vi "main.vi"() -> ()   [LabVIEW 2015]
uses:
  LabviewSubVI/RFConfig/RF_Config.ctl
  LabviewSubVI/RFConfig/StudentMsg.ctl
panel:
  out "信宿数据":dbl[](graph)
  out "信源数据":dbl[](graph)
  out "时隙同步相关峰":dbl[](graph)
  in  "相位纠正开关":enum16{"关", "开"}(ring)=enum."开"
  in  "载波调制开关":enum16{"关", "开"}(ring)=enum."开"
  in  "信道编码开关":enum16{"关", "开"}(ring)=enum."开"
  in  "解调载波初相位":enum16{"0", "180"}(ring) caption="下拉列表"
  in  "信噪比(dB)":dbl=40.0 caption="crc_num" min=-20.0 max=40.0 step=0.1 format="%#_13g"
  out "误码率":dbl format="%#_4g"
  out "误码数":dbl format="%#_13g"
  out "CRC\n校验结果":bool[](array[boolean])
  out "接收信号波形":dbl[](graph)
  in  "pcip":string="192.168.1.180"
  in  "xsrpip":string="192.168.1.166"
  out "发送信号波形":dbl[](graph)
  in  "运行方式":enum16{"仿真系统", "真实系统"}(ring)
  in  "?":T1={"发射频率"=2000000000, "发射衰减"=30, "接收频率"=2000000000, "接收增益"=22, "接收通道"=enum."RxCh1", "发射通道"=enum."TxCh1"} {"接收增益" max=40 format="%.0fdB"; "接收频率" min=70000000 max=6000000000 format="%.6pHz"; "发射衰减" max=90 format="%.0fdB"; "发射频率" min=70000000 max=6000000000 format="%.6pHz"}
  out "实验学生信息":T2={"姓名"="XXX\n", "学号"="XXX", "班级"="XXX", "学校"="XXX"}
  # "基于XSRP软件无线电平台的BPSK数字调制通信系统"
  # "实验参数设置"
  # "实验学生信息"
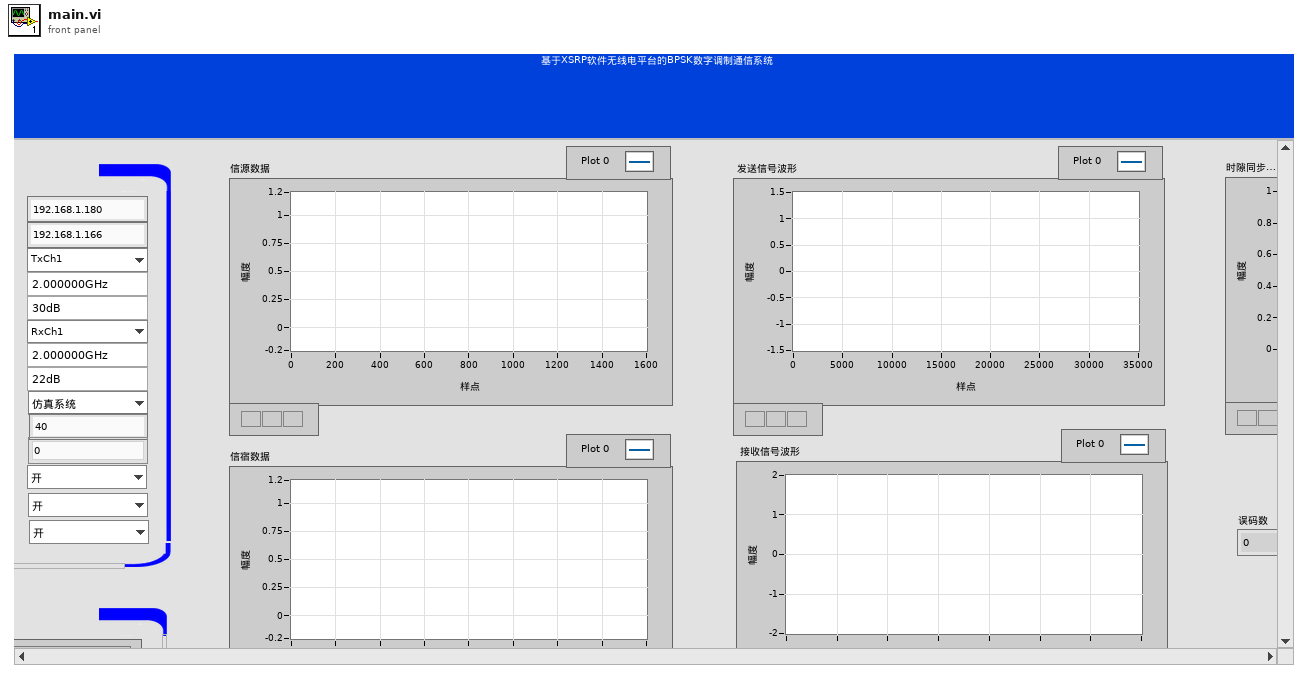
[diagram p1: front panel]
types:
  T1 = typedef "RF_Config.ctl" = cluster{"发射频率":u64, "发射衰减":u8, "接收频率":u64, "接收增益":u8, "接收通道":enum16{"RxCh1", "RxCh2"}, "发射通道":enum16{"TxCh1", "TxCh2"}}
  T2 = typedef "StudentMsg.ctl" = cluster{"姓名":string, "学号":string, "班级":string, "学校":string}
  T3 = enum8{"Enabled", "Disabled", "Disabled and Grayed Out"}
  T4 = cluster{"接收通道":enum16{"RxCh1", "RxCh2"}, "接收频率":u32, "接收增益":u8}
  T5 = cluster{"发射通道":enum16{"TxCh1", "TxCh2"}, "发射频率":u32, "发射衰减":u8}
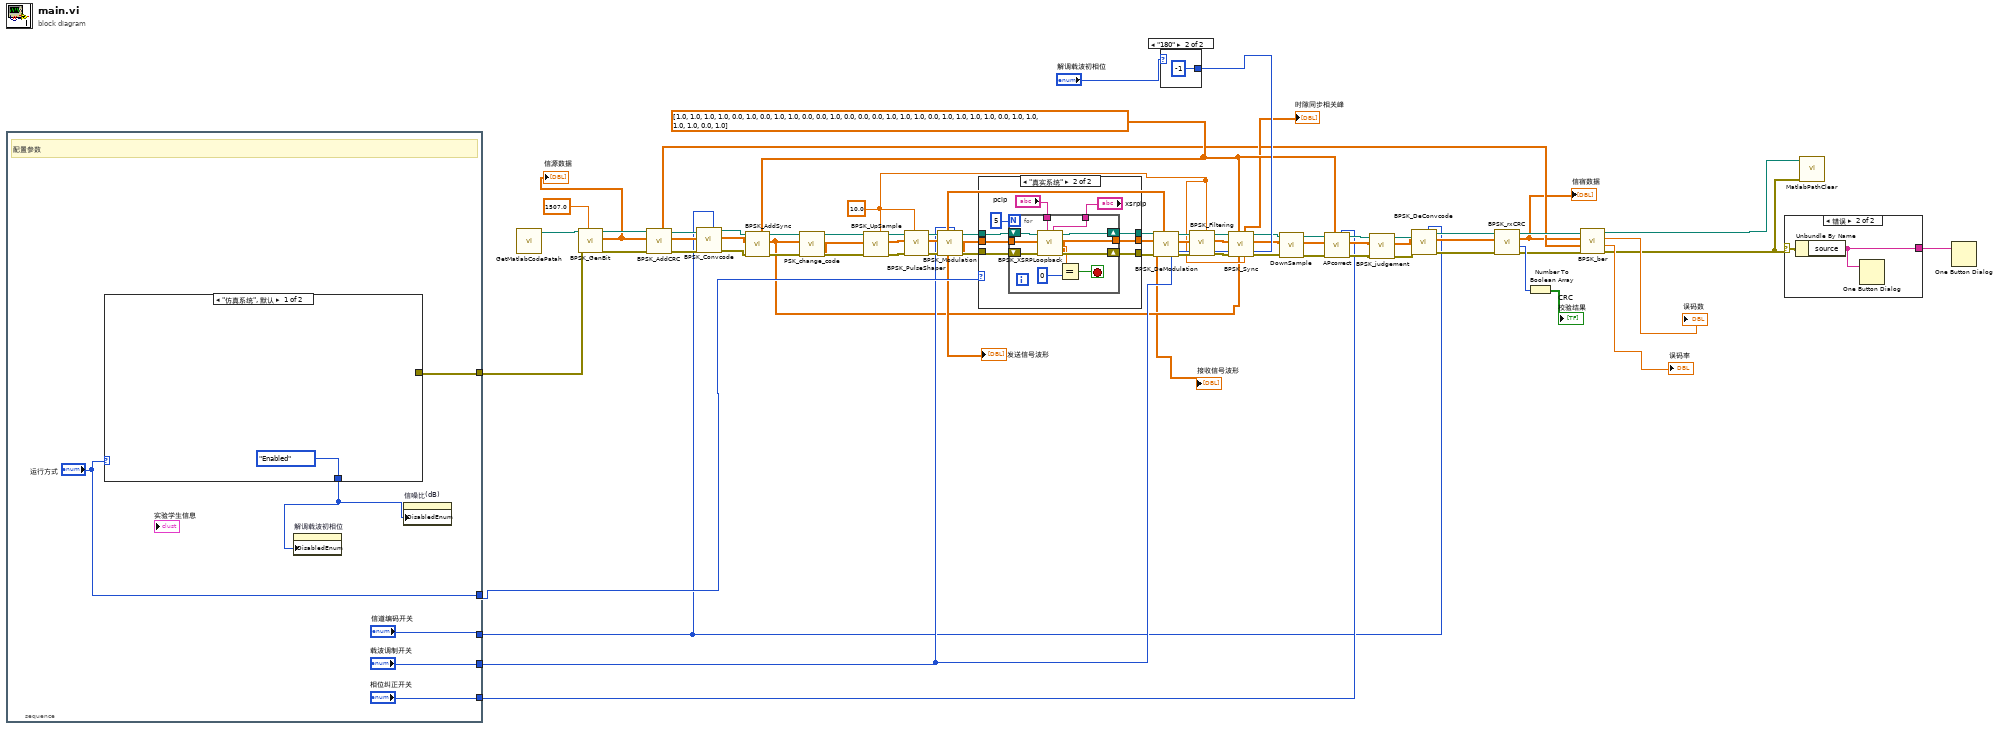
[diagram p0: block diagram]
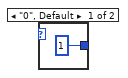
[diagram p2: hidden frame]
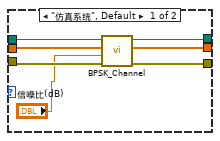
[diagram p3: hidden frame]
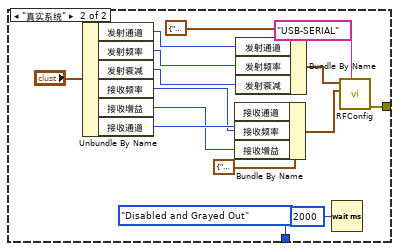
[diagram p4: hidden frame]
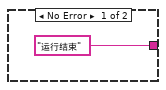
[diagram p5: hidden frame]
diagram:
  w8 = 10.0 ("UpSampleRate")
  w12 = dbl[] [1.0, 1.0, 1.0, 1.0, 0.0, 1.0, 0.0, 1.0, 1.0, 0.0, 0.0, 1.0, 0.0, 0.0, 0.0, 1.0, 1.0, 1.0, 0.0, 1.0, 1.0, 1.0, 1.0, 0.0, 1.0, 1.0, 1.0, 1.0, 0.0, 1.0] ("1-D Array of Real")
  n1 = stacked-sequence {
    tunnel: [w77] -> w33
    tunnel: ["运行方式"] -> w44
    tunnel: ["信道编码开关"] -> w9
    tunnel: ["载波调制开关"] -> w11
    tunnel: ["相位纠正开关"] -> w10
    frame #0 {
      # "配置参数"
      n2 = case shown="\"仿真系统\", 默认" "运行方式" {
        tunnel: [_ w82] -> w77
        tunnel: [T3."Enabled" ("Disabled") T3."Disabled and Grayed Out" ("Disabled")] -> w75
        frame "仿真系统", Default {
        }
        frame "真实系统" {
          n3 = Unbundle By Name("?") -> ("发射通道"=w90:enum16{"TxCh1", "TxCh2"}, "发射频率"=w89:u64, "发射衰减"=w88:u8, "接收频率"=w84:u64, "接收增益"=w85:u8, "接收通道"=w86:enum16{"RxCh1", "RxCh2"})
          n4 = Bundle By Name(cluster=T4 {"接收通道"=enum."RxCh1", "接收频率"=0, "接收增益"=0} ("接收参数设置"), "接收通道"=w86, "接收频率"=w84, "接收增益"=w85) -> (w83:T4)
          n5 = Bundle By Name(cluster=T5 {"发射通道"=enum."TxCh1", "发射频率"=0, "发射衰减"=0} ("发射参数设置"), "发射通道"=w90, "发射频率"=w89, "发射衰减"=w88) -> (w92:T5)
          n6 = Wait (ms)(milliseconds to wait=u32 2000) -> ()  [unwired: 1 out]
          n7 = call "RFConfig.vi"("USB-SERIAL name"="USB-SERIAL", "接收参数设置"=w83, "发射参数设置"=w92) -> ("error out"=w82:errorcluster)  [unwired: 8 in]
        }
      }
      n8 = property on="解调载波初相位" class="Enum (严格)"("DisabledEnum"=w75) -> ()  [unwired: 2 in, 2 out]
      n9 = property on="信噪比(dB)" class="DigNum (严格)"("DisabledEnum"=w75) -> ()  [unwired: 2 in, 2 out]
    }
  }
  n10 = call "GetMatlabCodePatah.vi"() -> ("MatlabCodePath"=w47:path)  [unwired: 11 in]
  n11 = call "BPSK_GenBit.vi"("MsgLen"=1507.0, "error in (no error)"=w33, "PathIn"=w47) -> ("error out"=w45:errorcluster, "SendBit"=w5:dbl[], "PathOut"=w46:path)  [unwired: 6 in]
  "信源数据" <- w5
  n12 = call "BPSK_AddCRC.vi"("error in (no error)"=w45, "input_data"=w5, "PathIn"=w46) -> ("error out"=w69:errorcluster, "output_data"=w68:dbl[], "PathOut"=w70:path)  [unwired: 6 in]
  n13 = call "BPSK_Convcode.vi"("EN_Convcode"=w9, "error in"=w69, "input_data"=w68, "Path In"=w70) -> ("error out"=w26:errorcluster, "output_data"=w25:dbl[], "Path Out"=w31:path)  [unwired: 5 in]
  n14 = call "BPSK_AddSync.vi"("Preamble"=w12, "error in (no error)"=w26, "Channel_Bit"=w25, "PathIn"=w31) -> ("error out"=w27:errorcluster, "data"=w3:dbl[], "PathOut"=w30:path)  [unwired: 5 in]
  n15 = call "PSK_change_code.vi"("error in (no error)"=w27, "input_data"=w3, "PathIn"=w30) -> ("error out"=w28:errorcluster, "PathOut"=w29:path, "x"=w6:dbl[])  [unwired: 6 in]
  n16 = call "BPSK_UpSample.vi"("UpSampleRate"=w8, "error in (no error)"=w28, "input_data"=w6, "PathIn"=w29) -> ("error out"=w57:errorcluster, "output_data"=w2:dbl[], "PathOut"=w58:path)  [unwired: 5 in]
  n17 = call "BPSK_PulseShaper.vi"("UpSampleRate"=w8, "error in (no error)"=w57, "input_data"=w2, "PathIn"=w58) -> ("error out"=w56:errorcluster, "out_data"=w34:dbl[], "PathOut"=w55:path)  [unwired: 5 in]
  n18 = call "BPSK_Modulation.vi"("EN_Modulation"=w11, "error in (no error)"=w56, "input_data"=w34, "PathIn"=w55) -> ("error out"=w53:errorcluster, "PathOut"=w54:path, "output_data"=w35:dbl[], "y"=w36:dbl[])  [unwired: 4 in]
  "发送信号波形" <- w35
  n19 = case shown="\"真实系统\"" w44 {
    tunnel: w54 -> [w98 w106]
    tunnel: w35 -> [w100 w102]
    tunnel: w53 -> [w99 w107]
    tunnel: [w97 w105] -> w52
    tunnel: [w96 w101] -> w1
    tunnel: [w95 w104] -> w51
    frame "仿真系统", Default {
      n20 = call "BPSK_Channel.vi"("error in (no error)"=w99, "snr"="信噪比(dB)", "txSig"=w100, "PathIn"=w98) -> ("error out"=w95:errorcluster, "rxSig"=w96:dbl[], "PathOut"=w97:path)  [unwired: 5 in]
    }
    frame "真实系统" {
      n21 = for {
        N: 5 -> [_]
        tunnel: "pcip" -> [w120]
        tunnel: "xsrpip" -> [w119]
        tunnel: [w110] -> w101
        shift-right: [w116] -> w104
        shift-left: w107 -> [w112]
        shift-right: [w117] -> w105
        shift-left: w106 -> [w118]
        tunnel: w102 -> [w111]
        stop <- w113 stop-if-true
        n22 = call "BPSK_XSRPLoopback.vi"("tx_data"=w111, "xsrpip"=w119, "pcip"=w120, "error in (no error)"=w112, "PathIn"=w118) -> ("error out"=w116:errorcluster, "ERR_CODE"=w114:dbl, "PathOut"=w117:path, "rxdataIQ"=w110:cdb[])  [unwired: 3 in]
        n23 = Equal?(x=w114, y=0) -> (x = y?=w113:bool)
      }
    }
  }
  "接收信号波形" <- w1
  n24 = case shown="\"180\"" "解调载波初相位" {
    tunnel: [1 -1] -> w38
    frame "0", Default {
    }
    frame "180" {
    }
  }
  n25 = call "BPSK_DeModulation.vi"("input_data"=w1, ",EN_Modulation"=w11, "ini_pha"=w38, "y"=w36, "error in (no error)"=w51, "PathIn"=w52) -> ("error out"=w50:errorcluster, "re_data"=w48:dbl[], "PathOut"=w49:path)  [unwired: 3 in]
  n26 = call "BPSK_Filtering.vi"("UpSampleRate"=w8, "error in (no error)"=w50, "input_data"=w48, "PathIn"=w49) -> ("error out"=w65:errorcluster, "out_data"=w66:dbl[], "PathOut"=w67:path)  [unwired: 5 in]
  n27 = call "BPSK_Sync.vi"("UpSampleRate"=w8, "data"=w3, "Preamble"=w12, "error in (no error)"=w65, "input_data"=w66, "PathIn"=w67) -> ("error out"=w18:errorcluster, "output_data"=w19:dbl[], "PathOut"=w22:path, "RecvCorr"=→"时隙同步相关峰":dbl[])  [unwired: 2 in]
  n28 = call "DownSample.vi"("error in (no error)"=w18, "input_data"=w19, "PathIn"=w22) -> ("error out"=w24:errorcluster, "out_data"=w17:dbl[], "PathOut"=w23:path)  [unwired: 6 in]
  n29 = call "APcorrect.vi"("EN_AP"=w10, "c"=w12, "error in"=w24, "inputData"=w17, "Path In"=w23) -> ("error out"=w14:errorcluster, "out_data"=w16:cdb[], "Path Out"=w21:path)  [unwired: 4 in]
  n30 = call "BPSK_judgement.vi"("error in (no error)"=w14, "input_data"=w16, "PathIn"=w21) -> ("error out"=w13:errorcluster, "judge_data"=w15:dbl[], "PathOut"=w20:path)  [unwired: 6 in]
  n31 = call "BPSK_DeConvcode.vi"("EN_Convcode"=w9, "error in"=w13, "inputData"=w15, "Path In"=w20) -> ("error out"=w64:errorcluster, "out_data"=w63:dbl[], "Path Out"=w62:path)  [unwired: 5 in]
  n32 = call "BPSK_rxCRC.vi"("error in (no error)"=w64, "input_data"=w63, "PathIn"=w62) -> ("error out"=w59:errorcluster, "CRC_flag"=w61:i32, "out_data"=w4:dbl[], "PathOut"=w60:path)  [unwired: 5 in]
  "信宿数据" <- w4
  n33 = Number To Boolean Array(number=w61) -> (Boolean array=→"CRC\n校验结果":bool[])
  n34 = call "BPSK_ber.vi"("error in"=w59, "rxbit"=w5, "txbit"=w4, "Path In"=w60) -> ("error out"=w39:errorcluster, "ber"=→"误码率":dbl, "errnum"=→"误码数":dbl, "Path Out"=w40:path)  [unwired: 4 in]
  n35 = case shown="错误" w39 {
    selector: w39 -> [_ w125]
    tunnel: ["运行结束" ("source") w124] -> w71
    frame No Error {
    }
    frame Error {
      n36 = Unbundle By Name(w125) -> ("source"=w124:string)
      n37 = One Button Dialog(message=w124) -> ()  [unwired: 1 in, 1 out]
    }
  }
  n38 = call "MatlabPathClear.vi"("error in"=w39, "Path"=w40) -> ()  [unwired: 9 in, 1 out]
  n39 = One Button Dialog(message=w71) -> ()  [unwired: 1 in, 1 out]
